vi "Exercise 1.2 - Mic Acquisition.vi"() -> ()   [LabVIEW 2024]
panel:
  out "Filtered Signal":dynamicdata(graph)
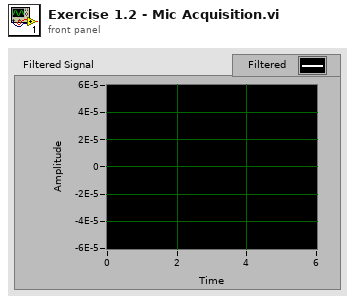
[diagram p1: front panel]
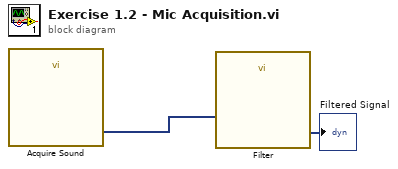
[diagram p0: block diagram]
diagram:
  n1 = call "Acquire Sound"() -> ("Data"=w1:dynamicdata)  [unwired: 18 in, 1 out]
  n2 = call "Filter"("Signal"=w1) -> ("Filtered Signal"=→"Filtered Signal":dynamicdata)  [unwired: 9 in, 1 out]
